vi "Relay (DBL Array).vi"(2 "initialize":bool, 3 "output when on/off":T1={"output when on"=1.0, "output when off"=0.0} {"output when off" format="%.2f"; "output when on" format="%.2f"}, 4 "switch on/off point":T2 {"switch off point" format="%.2f"; "switch on point" format="%.2f"}, 5 "Input Points":dbl[](array[numeric]) format="%.2f") -> (1 "Output Points":dbl[](array[numeric]) format="%.2f")   [LabVIEW 2017, in "NI_AdvCtrl_nonlinear.lvlib"]
doc: "LabVIEW no longer supports this VI. You can obtain similar functionality by installing the LabVIEW Simulation Module.\n\nSwitches between two constants. When the relay is on, it remains on until input drops below the value of switch off point. When the relay is off, it remains off until input exceeds the value of switch on point. The relay is predefined in the on state."
uses:
  <vilib>/addons/control/advanced/NI_AdvCtrl_nonlinear.lvlib
  <vilib>/addons/control/advanced/NI_AdvCtrl_continuous linear.lvlib
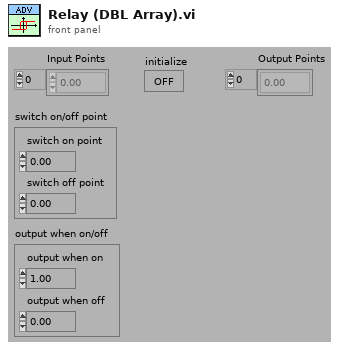
[diagram p1: front panel]
types:
  T1 = cluster{"output when on":dbl, "output when off":dbl}
  T2 = cluster{"switch on point":dbl, "switch off point":dbl}
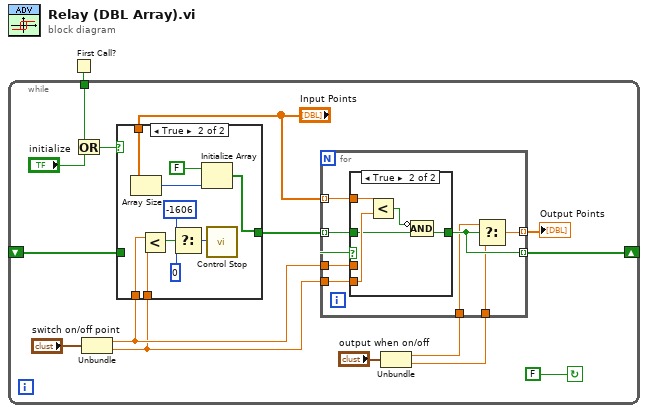
[diagram p0: block diagram]
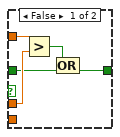
[diagram p2: hidden frame]
diagram:
  n1 = First Call?() -> (First Call?: T/F=w1:bool)
  n2 = while {
    tunnel: w1 -> [w12]
    shift-left: _ -> [w16]
    shift-right: [w10] -> _
    stop <- FALSE continue-if-true
    n3 = Or(x=w12, y="initialize") -> (x .or. y?=w13:bool)
    n4 = Unbundle("switch on/off point") -> ("switch on point"=w8:dbl, "switch off point"=w7:dbl)
    n5 = case shown="True" w13 {
      tunnel: w16 -> [w35 _]
      tunnel: [w35 w40] -> w15
      tunnel: w8 -> [_ w45]
      tunnel: w7 -> [_ w44]
      tunnel: "Input Points" -> [_ w41]
      frame False {
      }
      frame True {
        n6 = Array Size(array=w41) -> (size(s)=w43:i32)
        n7 = Less?(x=w45, y=w44) -> (x < y?=w37:bool)
        n8 = Select(t=-1606, s=w37, f=0) -> (s? t:f=w36:i32)
        n9 = Initialize Array(FALSE, w43) -> (w40:bool[])
        n10 = call <vilib>:"Control Stop.vi"("error"=w36) -> ()  [unwired: 2 out]
      }
    }
    n11 = Unbundle("output when on/off") -> ("output when on"=w4:dbl, "output when off"=w5:dbl)
    n12 = for {
      tunnel: "Input Points" -> [w24] mode=indexing
      tunnel: w15 -> [w23] mode=indexing
      tunnel: [w22] -> w2 mode=indexing
      tunnel: [w21] -> w10 mode=indexing
      tunnel: w8 -> [w20]
      tunnel: w7 -> [w19]
      tunnel: w5 -> [w18]
      tunnel: w4 -> [w17]
      n13 = case shown="True" w23 {
        tunnel: w24 -> [w29 w34]
        tunnel: w19 -> [_ w33]
        tunnel: w23 -> [w26 w31]
        tunnel: [w25 w30] -> w21
        tunnel: w20 -> [w28 _]
        frame False {
          n14 = Greater?(x=w29, y=w28) -> (0:w27:bool)
          n15 = Compound Arithmetic op=OR(w27, w26) -> (w25:bool)
        }
        frame True {
          n16 = Less?(x=w34, y=w33) -> (x < y?=w32:bool)
          n17 = Compound Arithmetic op=AND(invert w32, w31) -> (w30:bool)
        }
      }
      n18 = Select(t=w17, s=w21, f=w18) -> (s? t:f=w22:dbl)
    }
    "Output Points" <- w2
  }
